vi "Cond Timed Wait (absolute seconds).vi"(8 "error in (no error)":errorcluster, 9 "absolute timeout (seconds)":dbl, 10 "Mutex in":T1, 11 "Cond in":T2) -> (0 "error out":errorcluster, 1 "timed out?":bool, 2 "Mutex out":T1, 3 "Cond out":T2)   [LabVIEW 2013, in "Linux RT IPC.lvlib" / "POSIX Threads.lvlib" / "Cond.lvclass"]
doc: "Calls pthread_cond_timedwait() on the pthread cond object encapsulated by Cond.\n\nTo provide a valid absolute timeout, query the appropriate clock for the current time and offset the time by the desired timeout duration. By default, conditional variables use the Realtime clock when evaluating the absolute timeout, but this clock can be changed using the Cond attribute, Set Clock.\n\nRefer to online POSIX documentation for more information."
uses:
  Cond.lvclass
  Controls/reference.ctl
  Mutex/Controls/reference.ctl
  Mutex/Mutex.lvclass
  POSIX Thread Object/POSIX Thread Object.lvclass/POSIX Thread Object.ctl
  POSIX Thread Object/Private VIs/libpthread path.vi
  <vilib>/NI/NI Linux RT Utilities/VIs/Public/Convert Types/convert timespec 64 to timespec 32.vi
  POSIX Thread Object/Private VIs/get pthread error.vi
  POSIX Thread Object/POSIX Thread Object.lvclass
  <vilib>/NI/NI Linux RT Utilities/Linux RT Utilities.lvlib
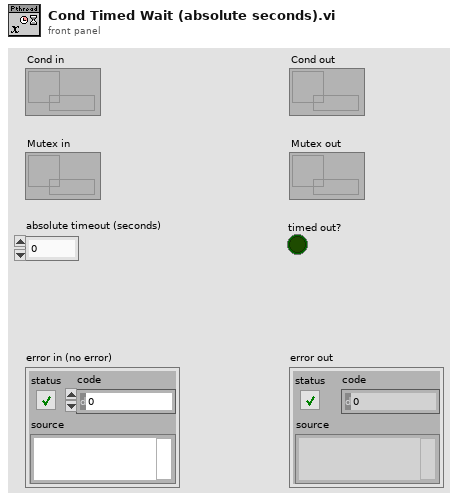
[diagram p1: front panel]
types:
  T1 = typedef "Linux RT IPC.lvlib/POSIX Threads.lvlib/Mutex.lvclass/reference.ctl" = refnum<data-value>
  T2 = typedef "Linux RT IPC.lvlib/POSIX Threads.lvlib/Cond.lvclass/reference.ctl" = refnum<data-value>
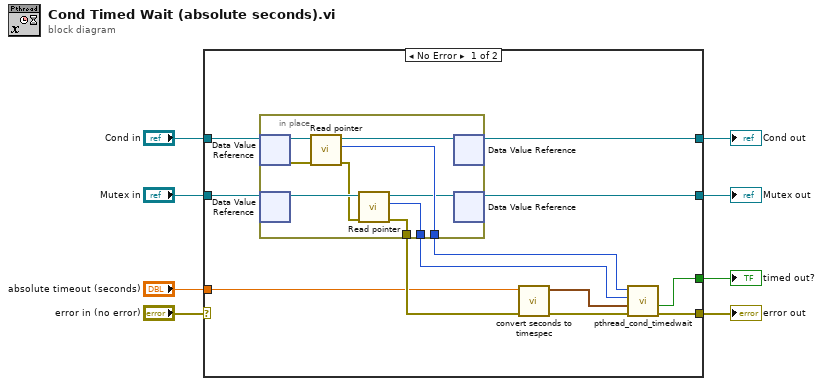
[diagram p0: block diagram]
diagram:
  n1 = case shown="No Error" "error in (no error)" {
    selector: "error in (no error)" -> [_ w31]
    tunnel: [w19 w31] -> w7
    tunnel: "Cond in" -> [w16 w30]
    tunnel: [w14 w30] -> w5
    tunnel: "Mutex in" -> [w15 w29]
    tunnel: [w13 w29] -> w3
    tunnel: "absolute timeout (seconds)" -> [w9 _]
    tunnel: [w18 _] -> w1
    frame No Error {
      n2 = in-place {
        in-place-border: [w25] -> w11
        in-place-border: [w21] -> w10
        in-place-border: [w20] -> w12
        n3 = in-place-dvr #1(w16) -> (w28:refnum<class "Cond.lvclass">, w26:errorcluster)
        n4 = in-place-dvr #2(w15) -> (w24:refnum<class "Mutex.lvclass">)  [unwired: 1 out]
        n5 = call "Read pointer.vi"("error in (no error)"=w26, "POSIX Thread Object in"=w28) -> ("error out"=w22:errorcluster, "pointer"=w25:u64, "POSIX Thread Object out"=w27:refnum<class "Cond.lvclass">)  [unwired: 7 in]
        n6 = call "Read pointer.vi"("error in (no error)"=w22, "POSIX Thread Object in"=w24) -> ("error out"=w21:errorcluster, "pointer"=w20:u64, "POSIX Thread Object out"=w23:refnum<class "Mutex.lvclass">)  [unwired: 7 in]
        n7 = in-place-dvr #1(w27) -> (w14:T2)  [unwired: 1 out]
        n8 = in-place-dvr #2(w23) -> (w13:T1)  [unwired: 1 out]
      }
      n9 = call <vilib>:"convert seconds to timespec.vi"("seconds"=w9) -> ("timespec"=w17:cluster{"sec":u64, "nsec":u64})  [unwired: 10 in]
      n10 = call "pthread_cond_timedwait.vi"("error in (no error)"=w10, "absolute time"=w17, "mutex ptr in"=w12, "cond ptr in"=w11) -> ("error out"=w19:errorcluster, "timed out?"=w18:bool)  [unwired: 4 in, 2 out]
    }
    frame Error {
    }
  }
  "Cond out" <- w5
  "error out" <- w7
  "Mutex out" <- w3
  "timed out?" <- w1
